vi "uTTA_GetCAL_Output.vi"(6 "Number of Samples":u32=10, 8 "error in":errorcluster, 9 "Timeout(ms)":i32=1000, 10 "RX Termination(\\n)":string="\n", 11 "VISA Refnum in":refnum<visa-resource-name>) -> (0 "error out":errorcluster, 1 "Temperatures":dbl[][](array[numeric]), 2 "ADCs":i32[][](array[numeric]), 3 "VISA Refnum out":refnum<visa-resource-name>, 4 "PGA":i32[](array[numeric]))   [LabVIEW 2021]
panel:
  out "String":string
  out "Received":string
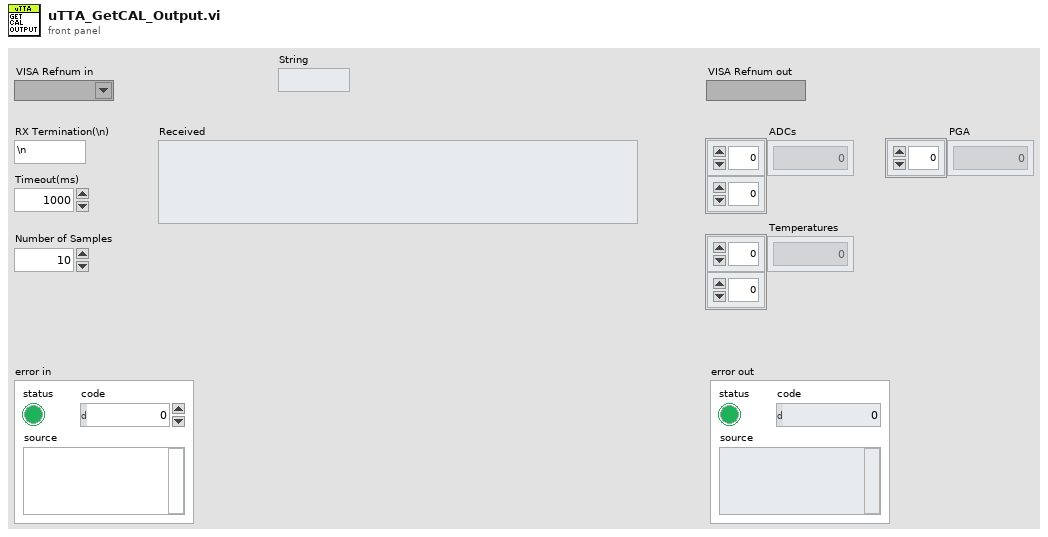
[diagram p1: front panel]
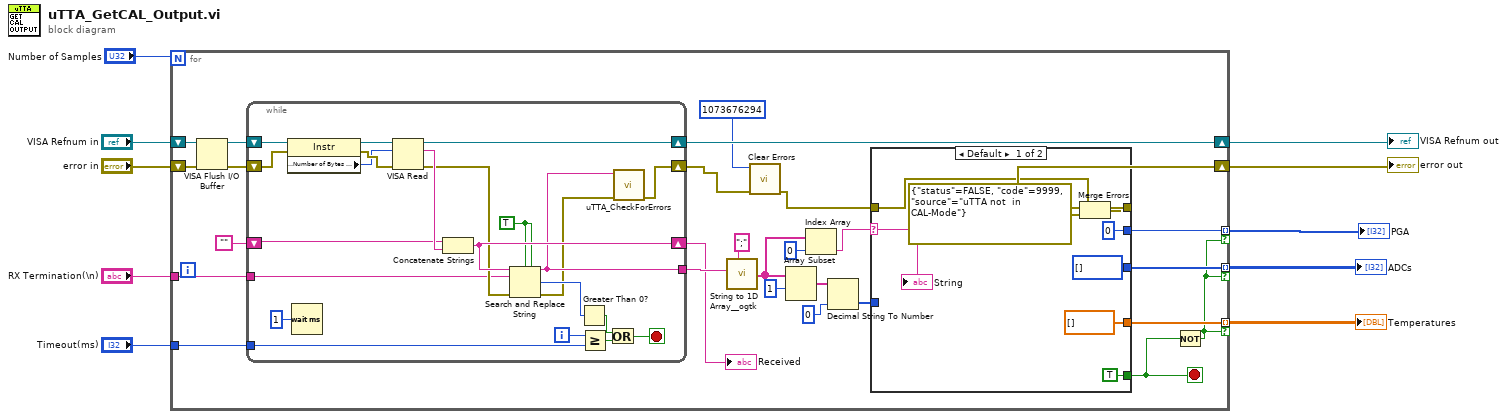
[diagram p0: block diagram]
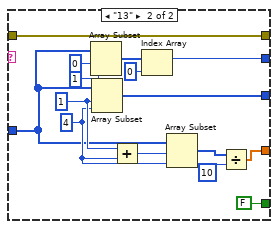
[diagram p2: hidden frame]
diagram:
  n1 = for {
    N: "Number of Samples" -> [_]
    tunnel: "RX Termination(\\n)" -> [w34]
    tunnel: "Timeout(ms)" -> [w33]
    tunnel: [w27] -> w3 mode=indexing if=w12
    tunnel: [w26] -> w2 mode=indexing if=w12
    shift-right: [w25] -> w7
    shift-left: "error in" -> [w37]
    shift-right: [w35] -> w8
    shift-left: "VISA Refnum in" -> [w36]
    tunnel: [w13] -> w1 mode=indexing if=w12
    stop <- w24 stop-if-true
    n2 = VISA Flush I/O Buffer(VISA resource name=w36, error in (no error)=w37) -> (VISA resource name out=w31:refnum<visa-resource-name>, error out=w30:errorcluster)  [unwired: 1 in]
    n3 = while {
      shift-right: [w75] -> w11
      shift-left: "" -> [w76]
      tunnel: [w64] -> w29
      shift-right: [w62] -> w22
      shift-left: w30 -> [w81]
      shift-right: [w72] -> w35
      shift-left: w31 -> [w82]
      tunnel: w33 -> [w66]
      tunnel: w34 -> [w65]
      i -> [w67]
      stop <- w69 stop-if-true
      w61 = TRUE ("ignore case? (F)")
      n4 = property class="Instr"(reference=w82, error in=w81) -> (reference out=w80:refnum<visa-resource-name>, error out=w79:errorcluster, "Serial Settings:Number of Bytes at Serial Port"=w78:u32)
      n5 = Wait (ms)(milliseconds to wait=u32 1) -> ()  [unwired: 1 out]
      n6 = VISA Read(VISA resource name=w80, byte count=w78, error in (no error)=w79) -> (VISA resource name out=w72:refnum<visa-resource-name>, read buffer=w77:string, error out=w71:errorcluster)  [unwired: 1 out]
      n7 = Concatenate Strings(w76, w77) -> (w75:string)
      n8 = Search and Replace String(case sensitive?=w61, multiline?=w61, input string=w75, search string=w65, error in=w71) -> (result string=w64:string, number of replacements=w74:i32, error out=w63:errorcluster)  [unwired: 3 in, 1 out]
      n9 = Greater Than 0?(x=w74) -> (x > 0?=w70:bool)
      n10 = Greater Or Equal?(x=w67, y=w66) -> (x >= y?=w68:bool)
      n11 = Or(x=w70, y=w68) -> (x .or. y?=w69:bool)
      n12 = call "uTTA_CheckForErrors.vi"("error in"=w63, "Received"=w64) -> ("error out"=w62:errorcluster)  [unwired: 9 in]
    }
    "Received" <- w11
    n13 = call <userlib>:"String to 1D Array__ogtk.vi"("delimiter (Tab)"=";", "string"=w29) -> ("Array of Strings"=w18:string[])  [unwired: 9 in]
    n14 = call <vilib>:"Clear Errors.vi"("error in (no error)"=w22, "specific error code to clear (0: all)"=1073676294) -> ("error out"=w21:errorcluster)  [unwired: 4 in, 1 out]
    n15 = Array Subset(array=w18, index=1) -> (w16:string[])  [unwired: 1 in]
    n16 = Index Array(array=w18, index=0) -> (element=w19:string)
    n17 = Decimal String To Number(string=w16, default (0L)=0 ("default (0 I32)")) -> (number=w14:i32[])  [unwired: 1 in, 1 out]
    n18 = case shown="Default" w19 {
      selector: w19 -> [w38 _]
      tunnel: [i32[] [] w58] -> w27
      tunnel: [dbl[] [] w56] -> w26
      tunnel: w21 -> [w43 w60]
      tunnel: [w44 w60] -> w25
      tunnel: [TRUE FALSE] -> w24
      tunnel: w14 -> [_ w51]
      tunnel: [0 w47] -> w13
      frame Default {
        n19 = Merge Errors(w43, errorcluster {"status"=FALSE, "code"=9999, "source"="uTTA not  in CAL-Mode"} ("error in")) -> (w44:errorcluster)
        "String" <- w38
      }
      frame "13" {
        w52 = 4 ("length")
        w54 = 1 ("index")
        n20 = Array Subset(array=w51, index=0, length=1) -> (w48:i32[])
        n21 = Array Subset(array=w51, index=w54, length=w52) -> (w58:i32[])
        n22 = Add(x=w54, y=w52) -> (x+y=w53:i32)
        n23 = Index Array(array=w48, index=0) -> (element=w47:i32)
        n24 = Array Subset(array=w51, index=w53, length=w52) -> (w57:i32[])
        n25 = Divide(x=w57, y=10) -> (x/y=w56:dbl[])
      }
    }
    n26 = Not(x=w24) -> (.not. x?=w12:bool)
  }
  "VISA Refnum out" <- w8
  "error out" <- w7
  "ADCs" <- w3
  "Temperatures" <- w2
  "PGA" <- w1
